vi "FilterChannelData.vi"(8 "error in (no error)":errorcluster, 11 "EMG in":refnum<class "EMG.lvclass">) -> (0 "error out":errorcluster, 2 "Filtered EMG":dbl[][](graph), 3 "EMG out":refnum<class "EMG.lvclass">)   [LabVIEW 2015, in "EMG.lvclass"]
uses:
  EMG.lvclass
  EMG.lvclass/EMG.ctl
  <vilib>/Analysis/3filter.llb/Filter Passband Type.ctl
  CustomVIs/CustomVI.lvlib
  <vilib>/Analysis/NI_AALBase.lvlib
panel:
  out "Filtered EMG 3":dbl[][](graph)
  out "Filtered EMG 2":dbl[][](graph)
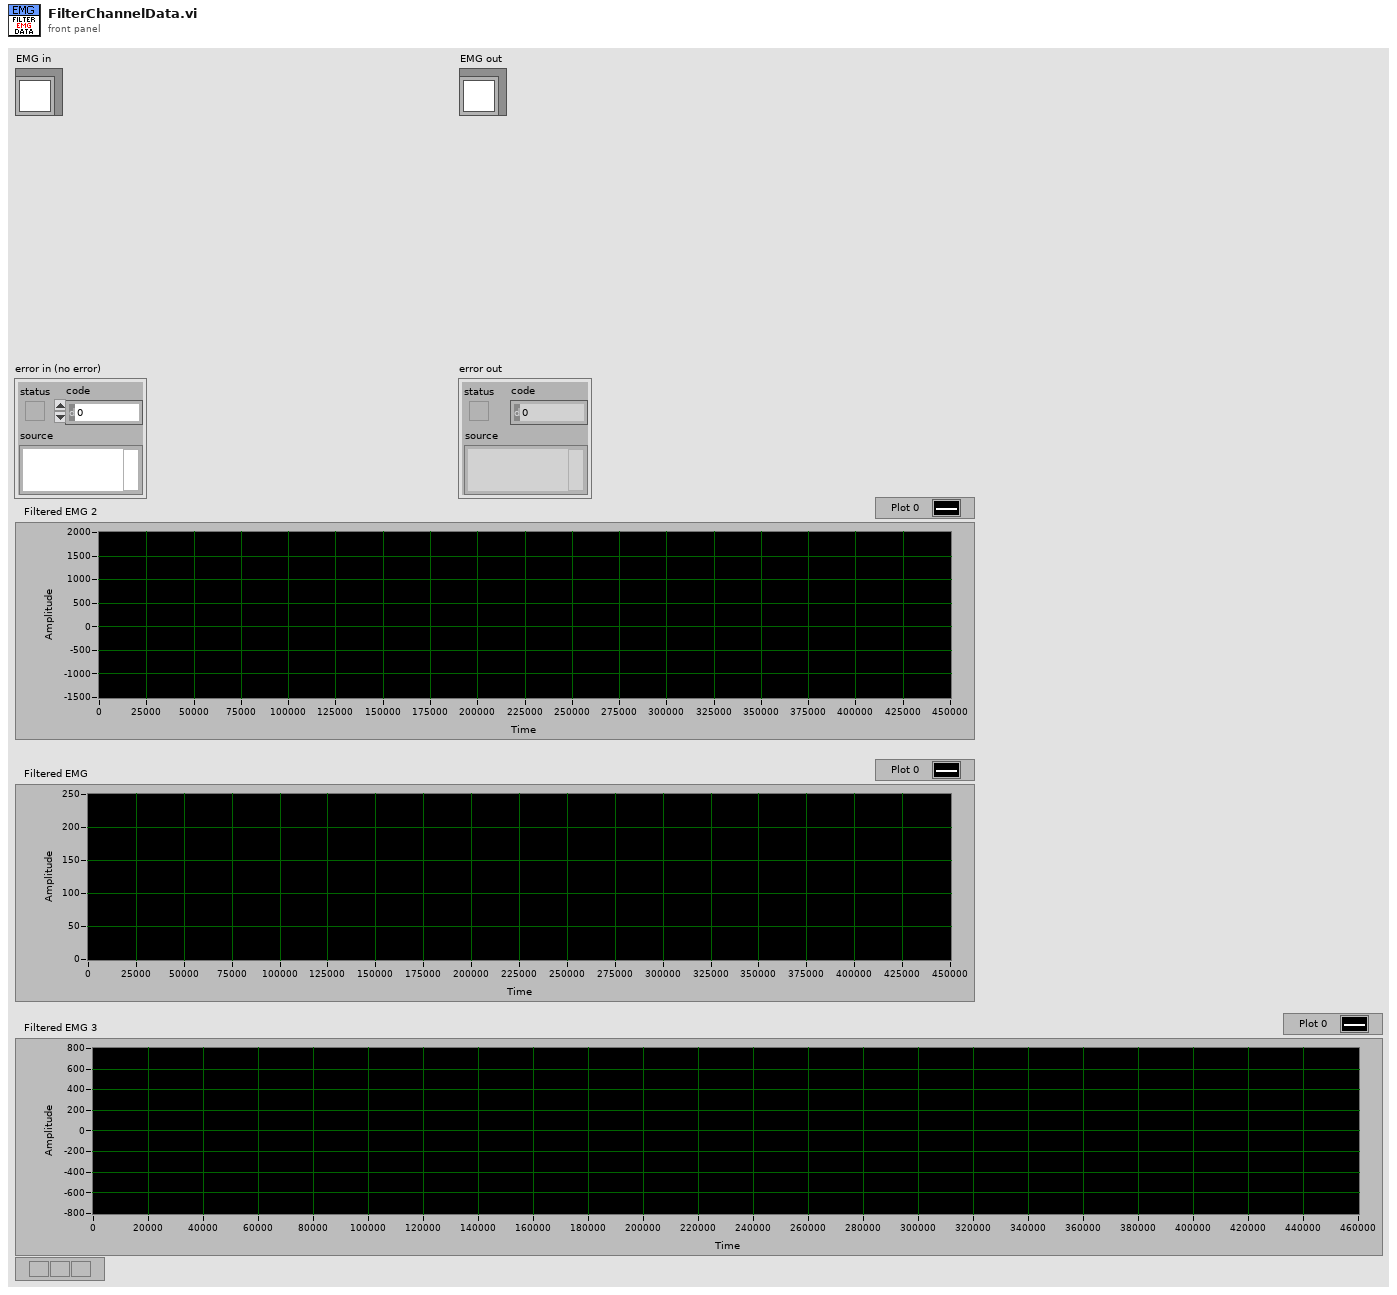
[diagram p1: front panel]
types:
  T1 = typedef "NI_AALBase.lvlib/Filter Passband Type.ctl" = enum32{"Lowpass", "Highpass", "Bandpass", "Bandstop"}
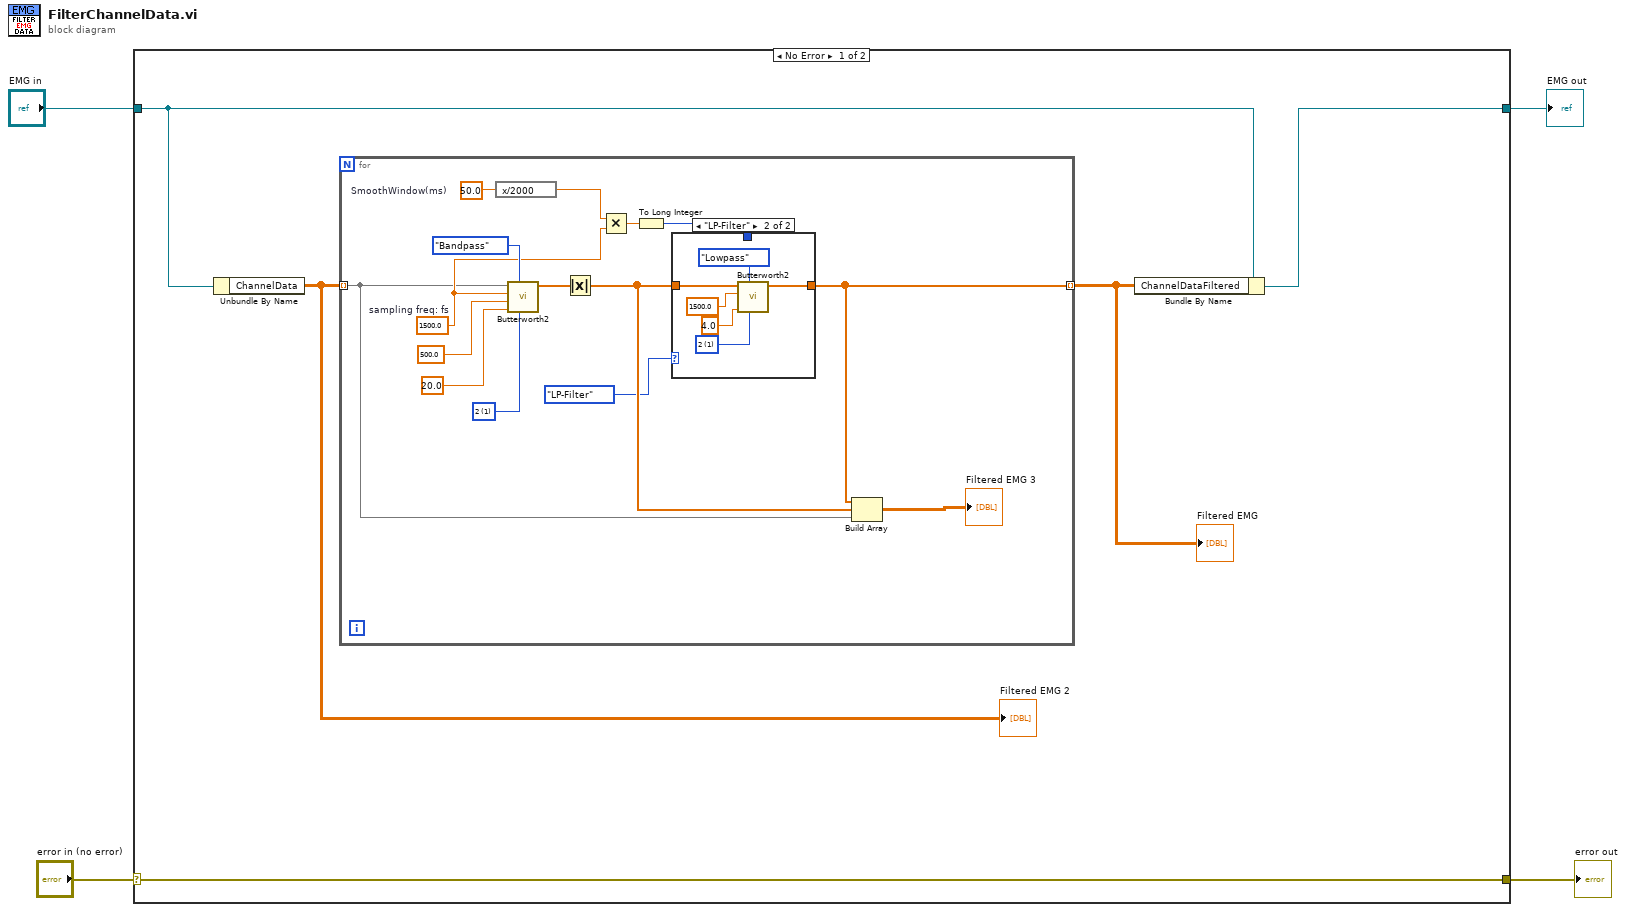
[diagram p0: block diagram]
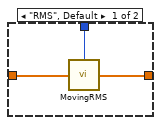
[diagram p2: hidden frame]
diagram:
  n1 = case shown="No Error" "error in (no error)" {
    selector: "error in (no error)" -> [w9 w35]
    tunnel: [w9 w35] -> w3
    tunnel: [w7 w34] -> w1
    tunnel: "EMG in" -> [w8 w34]
    frame No Error {
      n2 = Unbundle By Name(w8) -> ("ChannelData"=w5:dbl[][])
      "Filtered EMG 2" <- w5
      n3 = for {
        tunnel: w5 -> [w14] mode=indexing
        tunnel: [w12] -> w6 mode=indexing
        w19 = 50.0  # SmoothWindow(ms)
        w21 = u16 1 items=["2"=1, "4"=2, "6"=3, "8"=4, "10"=5] ("Order")
        w18 = 1500.0  # sampling freq: fs
        n4 = expression code="x/2000"(w19) -> (w17:dbl)
        n5 = call "Butterworth2.vi"("Order"=w21, "filter type"=Filter_Passband_Type."Bandpass", "low cutoff freq: fl"=20.0, "high cutoff freq: fh"=500.0, "sampling freq: fs"=w18, "X"=w14) -> ("Filtered X"=w20:dbl[])  [unwired: 5 in]
        n6 = Absolute Value(x=w20) -> (abs(x)=w11:dbl[])
        n7 = Multiply(x=w17, y=w18) -> (x*y=w16:dbl)
        n8 = To Long Integer(number=w16) -> (32bit integer=w15:i32)
        n9 = case shown="\"LP-Filter\"" enum16{"RMS", "LP-Filter"}."LP-Filter" {
          tunnel: w15 -> [w27 _]
          tunnel: [w26 w32] -> w12
          tunnel: w11 -> [w25 w33]
          frame "RMS", Default {
            n10 = call "MovingRMS.vi"("Half Window"=w27, "Array in"=w25) -> ("Array out"=w26:dbl[])  [unwired: 2 in]
          }
          frame "LP-Filter" {
            w29 = u16 1 items=["2"=1, "4"=2, "6"=3, "8"=4, "10"=5] ("Order")
            n11 = call "Butterworth2.vi"("Order"=w29, "filter type"=Filter_Passband_Type."Lowpass", "low cutoff freq: fl"=4.0, "sampling freq: fs"=1500.0, "X"=w33) -> ("Filtered X"=w32:dbl[])  [unwired: 6 in]
          }
        }
        n12 = Build Array(w12, w11, w14) -> (→"Filtered EMG 3":dbl[][])
      }
      "Filtered EMG" <- w6
      n13 = Bundle By Name(cluster=w8, "ChannelDataFiltered"=w6) -> (w7:refnum<class "EMG.lvclass">)
    }
    frame Error {
    }
  }
  "error out" <- w3
  "EMG out" <- w1
